vi "Timer_With_Stop_button.vi"(6 "Action (Time Elapsed)":T1=enum."TimeElapsed", 8 "error in (no error)":errorcluster, 11 "Time To Elapse":dbl) -> (0 "error out":errorcluster, 1 "Time Elapsed?":bool, 3 "Time Elapsed (s)":dbl)   [LabVIEW 2022 SP3]
doc: "This VI checks whether the Elapsed Time has Elapsed"
uses:
  #typedef_TimerAction.ctl
panel:
  out "Time To Elapse After Stop":dbl
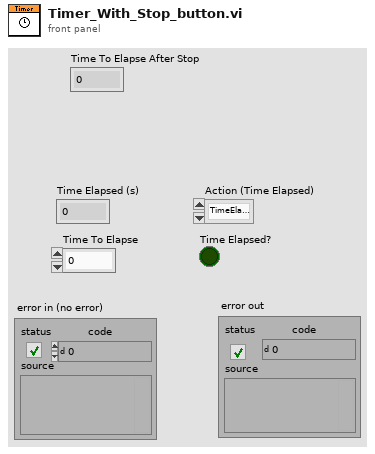
[diagram p1: front panel]
types:
  T1 = typedef "#typedef_TimerAction.ctl" = enum16{"Stop", "Reset", "TimeElapsed"}
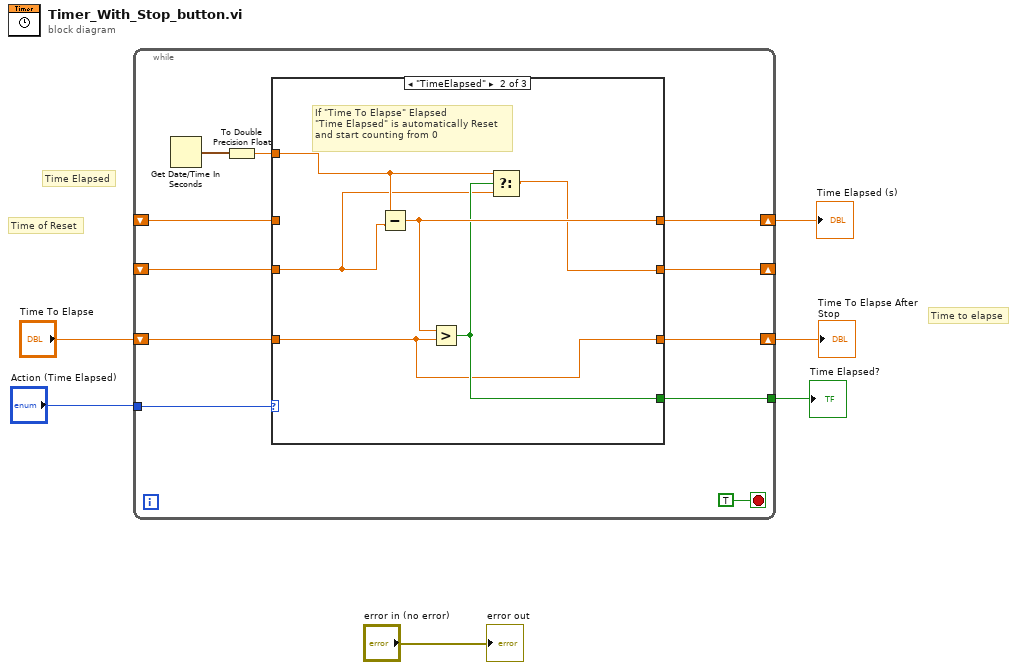
[diagram p0: block diagram]
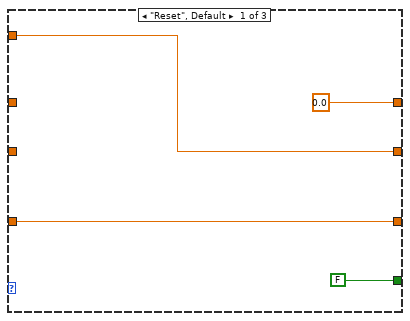
[diagram p2: hidden frame]
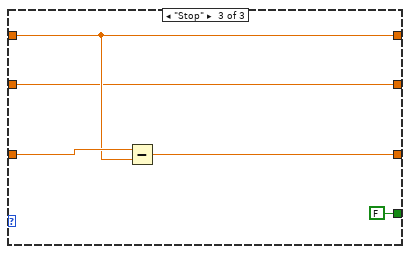
[diagram p3: hidden frame]
diagram:
  # "Time Elapsed"
  # "Time to elapse"
  # "Time of Reset"
  n1 = while {
    shift-right: [w13] -> _
    shift-left: _ -> [w12]
    tunnel: "Action (Time Elapsed)" -> [w16]
    tunnel: [w9] -> w2
    shift-right: [w11] -> w5
    shift-left: _ -> [w8]
    shift-right: [w7] -> w1
    shift-left: "Time To Elapse" -> [w10]
    stop <- TRUE stop-if-true
    n2 = Get Date/Time In Seconds() -> (seconds since 1Jan1904=w15:timestamp)
    n3 = To Double Precision Float(number=w15) -> (double precision float=w14:dbl)
    n4 = case shown="\"TimeElapsed\"" w16 {
      tunnel: w14 -> [w21 w25 _]
      tunnel: [w21 w23 w29] -> w13
      tunnel: w12 -> [_ w24 w29]
      tunnel: [0.0 w27 w30] -> w11
      tunnel: w10 -> [w18 w22 w32]
      tunnel: [FALSE w26 FALSE] -> w9
      tunnel: w8 -> [_ _ w30]
      tunnel: [w18 w22 w31] -> w7
      frame "Reset", Default {
      }
      frame "TimeElapsed" {
        # "If \"Time To Elapse\" Elapsed\n\"Time Elapsed\" is automatically Reset\nand start counting from 0"
        n5 = Subtract(x=w25, y=w24) -> (x-y=w27:dbl)
        n6 = Greater?(x=w27, y=w22) -> (0:w26:bool)
        n7 = Select(t=w25, s=w26, f=w24) -> (s? t:f=w23:dbl)
      }
      frame "Stop" {
        n8 = Subtract(x=w32, y=w30) -> (x-y=w31:dbl)
      }
    }
  }
  "Time Elapsed (s)" <- w5
  "Time Elapsed?" <- w2
  "Time To Elapse After Stop" <- w1
  "error out" <- "error in (no error)"
